vi "VisionAlign.vi"(6 "Offset":dbl=2.5, 8 "Error In":errorcluster, 10 "Setpoint":dbl=15.0) -> (0 "Error Out":errorcluster)   [LabVIEW 2016]
uses:
  <vilib>/addons/control/pid/NI_PID_pid.lvlib
  <vilib>/addons/control/pid/pid.llb/PID (DBL).vi
  <vilib>/Rock Robotics/Network Tables/NT Read Number.vi
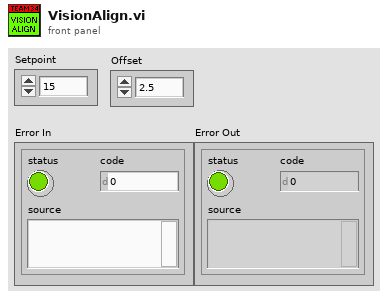
[diagram p1: front panel]
types:
  T1 = cluster{"proportional gain (Kc)":dbl, "integral time (Ti, min)":dbl, "derivative time (Td, min)":dbl}
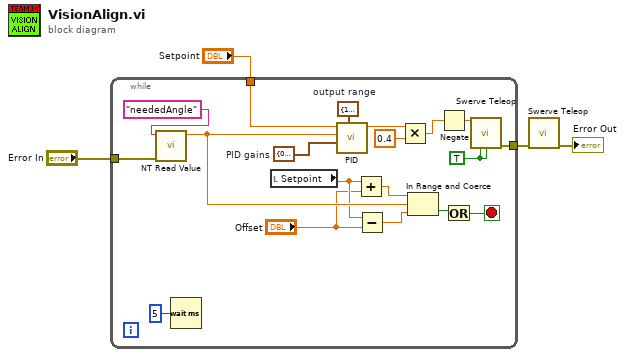
[diagram p0: block diagram]
diagram:
  n1 = while {
    tunnel: [w21] -> w4
    tunnel: "Error In" -> [w15]
    tunnel: "Setpoint" -> [w9]
    stop <- w14 stop-if-true
    w17 = cluster{"output high":dbl, "output low":dbl} {"output high"=1.0, "output low"=-1.0}  # output range
    w18 = T1 {"proportional gain (Kc)"=0.04, "integral time (Ti, min)"=0.0, "derivative time (Td, min)"=0.0}  # PID gains
    w20 = TRUE ("Robot Centric?")
    n2 = call-poly <vilib>:"NT Read Value.vi"("error in"=w15, "Name"="neededAngle") -> ("Numeric"=w10:dbl)  [unwired: 8 in, 1 out]
    n3 = Wait (ms)(milliseconds to wait=u32 5) -> ()  [unwired: 1 out]
    n4 = local read "Setpoint"() -> (w7:dbl)
    n5 = call-poly <vilib>:"PID.vi"("output range"=w17, "PID gains"=w18, "process variable"=w10, "setpoint"=w9) -> ("output"=w23:dbl)  [unwired: 6 in, 1 out]
    n6 = Add(x=w7, y="Offset") -> (x+y=w8:dbl)
    n7 = Subtract(x=w7, y="Offset") -> (x-y=w5:dbl)
    n8 = Multiply(x=w23, y=0.4) -> (x*y=w12:dbl)
    n9 = In Range and Coerce(upper limit=w8, x=w10, lower limit=w5) -> (In Range?=w13:bool)  [unwired: 1 out]
    n10 = Negate(x=w12) -> (-x=w11:dbl)
    n11 = Or(x=w13) -> (x .or. y?=w14:bool)  [unwired: 1 in]
    n12 = call "Swerve Teleop.vi"("X"=w11, "Robot Centric?"=w20, "Autonomous?"=w20) -> ("Error Out"=w21:errorcluster)  [unwired: 8 in, 4 out]
  }
  n13 = call "Swerve Teleop.vi"("Error In"=w4) -> ("Error Out"=→"Error Out":errorcluster)  [unwired: 10 in, 4 out]
